vi "Main.Create XNET Data Sessions.vi"(6 "Data":T1 {"Outgoing"."Trigger.Refs"."Data Reference" format="%.0x"; "Outgoing"."Disable.Refs"."Data Reference" format="%.0x"; "Outgoing"."Data.Refs"."Data Reference" format="%.0x"; "Incoming"."Timing.Refs"."Data Reference" format="%.0x"; "Incoming"."Data.Refs"."Data Reference" format="%.0x"}, 8 "error in (no error)":errorcluster, 9 "Network":T16 {"Name" format="%.0x"}, 10 "J1939 XNET Settings":T17 {"Termination" items=["Off", "On"]}, 11 "DataTableLUT":variant) -> (0 "error out":errorcluster, 2 "XNET Sessions":T18 {"Outgoing.Frames.CountersAndProtections"."Protection Configurations"."CRC Channels"."Data Type" items=["Signed", "Unsigned", "IEEE Float"]; "Trigger.Refs"."Data Reference" format="%.0x"; "Disable.Refs"."Data Reference" format="%.0x"; "Timing.Refs"."Data Reference" format="%.0x"; "Network"."Name" format="%.0x"; "Incoming.Refs"."Data Reference" format="%.0x"; "Outgoing.Refs"."Data Reference" format="%.0x"}, 3 "DataTableLUT":variant)   [LabVIEW 2021, in "J1939 Addon Engine.lvlib"]
uses:
  J1939 Addon Engine.lvlib
  Types/Protocol.XNET Refs.ctl
  Addon Shared/Types/Monitor Settings.ctl
  <vilib>/NI VeriStand/Custom Device API/Block Data Reference.ctl
  <vilib>/NI VeriStand/Custom Device API/Data Reference.ctl
  Types/Main.Outgoing.Frame.Settings.ctl
  Addon Shared/Types/Outgoing Event Trigger Types.ctl
  SubModules/Frame-Protection-Support/Source/Shared/Types/Exported Frame Settings.ctl
  SubModules/Frame-Protection-Support/Source/Shared/Types/Exported Frame Type.ctl
  SubModules/Frame-Protection-Support/Source/Shared/Types/Exported Protection Settings.ctl
  SubModules/Frame-Protection-Support/Source/Shared/Types/Protection Type.ctl
  SubModules/Frame-Protection-Support/Source/Shared/Types/XNET Signal Configuration.ctl
  SubModules/Frame-Protection-Support/Source/Shared/Types/Exported Counter Settings.ctl
  SubModules/Frame-Protection-Support/Source/Shared/Types/Exported Event Trigger Type.ctl
  Addon Shared/Types/XNET Settings.ctl
  Addon Shared/Types/Device Settings.ctl
  Addon Shared/Types/Incoming Settings.ctl
  Addon Shared/Types/Incoming Frame Settings.ctl
  Addon Shared/Types/Outgoing Settings.ctl
  Addon Shared/Types/Outgoing Frame Settings.ctl
  <vilib>/xnet/xnet.llb/XNET Control Scope.ctl
  Support Libraries/J1939 Utilities/SubVIs/Convert CAN Arb ID to J1939 ID.vi
  <vilib>/xnet/xnet.llb/XNET Create Session (Signal Input Single-point).vi
  <vilib>/xnet/xnet.llb/XNET Create Session (Signal Output Single-point).vi
  <resource>/objmgr/xnet.rc
  <vilib>/NI VeriStand/Custom Device API/Custom Device API.lvlib
  Addon Shared/J1939 Addon Shared.lvlib
  SubModules/Frame-Protection-Support/Source/Shared/Protection and Counter Support Shared.lvlib
  Support Libraries/J1939 Utilities/J1939 Utilities.lvlib
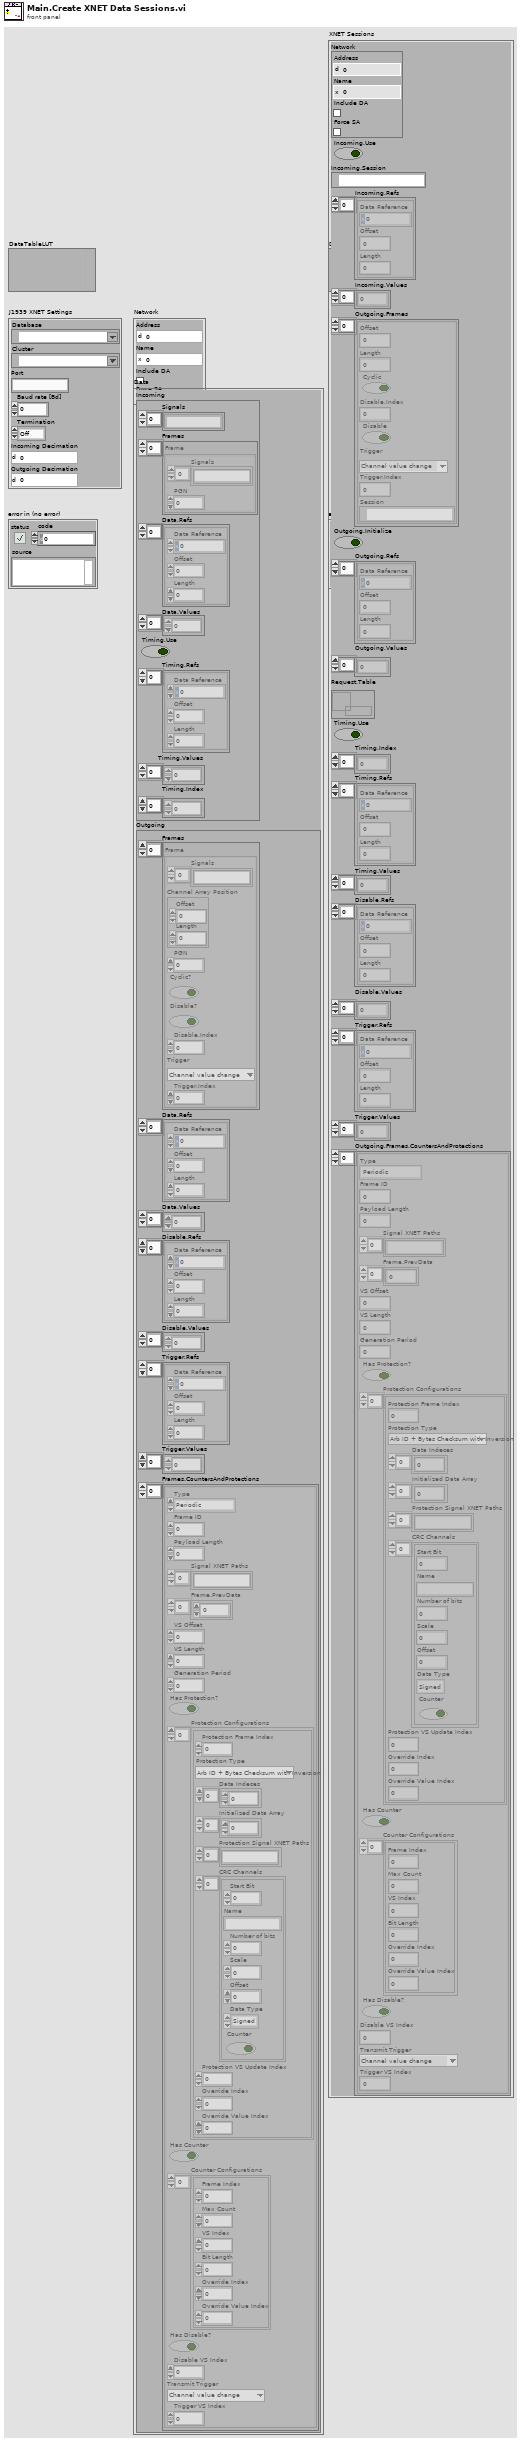
[diagram p1: front panel]
types:
  T1 = typedef "J1939 Addon Shared.lvlib/Device Settings.ctl" = cluster{"Incoming":T2, "Outgoing":T6}
  T2 = typedef "J1939 Addon Shared.lvlib/Incoming Settings.ctl" = cluster{"Signals":string[], "Frames":T3[], "Data.Refs":T4[], "Data.Values":dbl[], "Timing.Use":bool, "Timing.Refs":T4[], "Timing.Values":dbl[], "Timing.Index":i32[]}
  T3 = typedef "J1939 Addon Shared.lvlib/Incoming Frame Settings.ctl" = cluster{"Signals":string[], "PGN":u32}
  T4 = typedef "Custom Device API.lvlib/Block Data Reference.ctl" = cluster{"Data Reference":T5, "Offset":u64, "Length":u64}
  T5 = typedef "Custom Device API.lvlib/Data Reference.ctl" = i32
  T6 = typedef "J1939 Addon Shared.lvlib/Outgoing Settings.ctl" = cluster{"Frames":T7[], "Data.Refs":T4[], "Data.Values":dbl[], "Disable.Refs":T4[], "Disable.Values":dbl[], "Trigger.Refs":T4[], "Trigger.Values":dbl[], "Frames.CountersAndProtections":T9[]}
  T7 = typedef "J1939 Addon Shared.lvlib/Outgoing Frame Settings.ctl" = cluster{"Signals":string[], "Channel Array Position":cluster{"Offset":u32, "Length":u32}, "PGN":u32, "Cyclic?":bool, "Disable?":bool, "Disable.Index":i32, "Trigger":T8, "Trigger.Index":i32}
  T8 = typedef "J1939 Addon Shared.lvlib/Outgoing Event Trigger Types.ctl" = enum16{"Channel value change", "Trigger channel (not zero)", "Channel value change or trigger channel (not zero)", "Trigger channel (any value change)", "Channel value change or trigger channel (any value change)"}
  T9 = typedef "Protection and Counter Support Shared.lvlib/Exported Frame Settings.ctl" = cluster{"Type":T10, "Frame ID":u32, "Payload Length":u32, "Signal XNET Paths":string[], "Frame.PrevData":dbl[], "VS Offset":i32, "VS Length":i32, "Generation Period":u32, "Has Protection?":bool, "Protection Configurations":T11[], "Has Counter":bool, "Counter Configurations":T14[], "Has Disable?":bool, "Disable VS Index":i32, "Transmit Trigger":T15, "Trigger VS Index":i32}
  T10 = typedef "Protection and Counter Support Shared.lvlib/Exported Frame Type.ctl" = enum16{"Periodic", "Event", "Periodic/Event"}
  T11 = typedef "Protection and Counter Support Shared.lvlib/Exported Protection Settings.ctl" = cluster{"Protection Frame Index":i32, "Protection Type":T12, "Data Indeces":i32[], "Initialized Data Array":dbl[], "Protection Signal XNET Paths":string[], "CRC Channels":T13[], "Protection VS Update Index":i32, "Override Index":i32, "Override Value Index":i32}
  T12 = typedef "Protection and Counter Support Shared.lvlib/Protection Type.ctl" = enum16{"Arb ID + Bytes Checksum with Inversion", "Arb ID + Bytes CRC with Inversion", "Reversed Raw Signal Checksum with Inversion", "Concatenated Two's Compliment"}
  T13 = typedef "Protection and Counter Support Shared.lvlib/XNET Signal Configuration.ctl" = cluster{"Start Bit":i32, "Name":string, "Number of bits":i32, "Scale":dbl, "Offset":dbl, "Data Type":u32, "Counter":bool}
  T14 = typedef "Protection and Counter Support Shared.lvlib/Exported Counter Settings.ctl" = cluster{"Frame Index":i32, "Max Count":dbl, "VS Index":i32, "Bit Length":i64, "Override Index":i32, "Override Value Index":i32}
  T15 = typedef "Protection and Counter Support Shared.lvlib/Exported Event Trigger Type.ctl" = enum16{"Channel value change", "Trigger channel (not zero)", "Channel value change or trigger channel (not zero)", "Trigger channel (any value change)", "Channel value change or trigger channel (any value change)"}
  T16 = typedef "J1939 Addon Shared.lvlib/Monitor Settings.ctl" = cluster{"Address":u8, "Name":u64, "Include DA":bool, "Force SA":bool}
  T17 = typedef "J1939 Addon Shared.lvlib/XNET Settings.ctl" = cluster{"Database":refnum<k21>, "Cluster":refnum<k21>, "Port":string, "Baud rate [Bd]":u32, "Termination":u32, "Incoming Decimation":u32, "Outgoing Decimation":u32}
  T18 = typedef "J1939 Addon Engine.lvlib/Protocol.XNET Refs.ctl" = cluster{"Network":T16, "Incoming.Use":bool, "Incoming.Session":refnum<k21>, "Incoming.Refs":T4[], "Incoming.Values":dbl[], "Outgoing.Frames":T19[], "Outgoing.Initialize":bool, "Outgoing.Refs":T4[], "Outgoing.Values":dbl[], "Request.Table":refnum<k33>, "Timing.Use":bool, "Timing.Index":i32[], "Timing.Refs":T4[], "Timing.Values":dbl[], "Disable.Refs":T4[], "Disable.Values":dbl[], "Trigger.Refs":T4[], "Trigger.Values":dbl[], "Outgoing.Frames.CountersAndProtections":T9[]}
  T19 = typedef "J1939 Addon Engine.lvlib/Main.Outgoing.Frame.Settings.ctl" = cluster{"Offset":u32, "Length":u32, "Cyclic":bool, "Disable.Index":i32, "Disable":bool, "Trigger":T8, "Trigger.Index":i32, "Session":refnum<k21>}
  T20 = cluster{"read mode":enum16{"polling", "blocking"}, "write mode":enum16{"polling", "blocking"}}
  T21 = typedef "XNET Control Scope.ctl" = u32
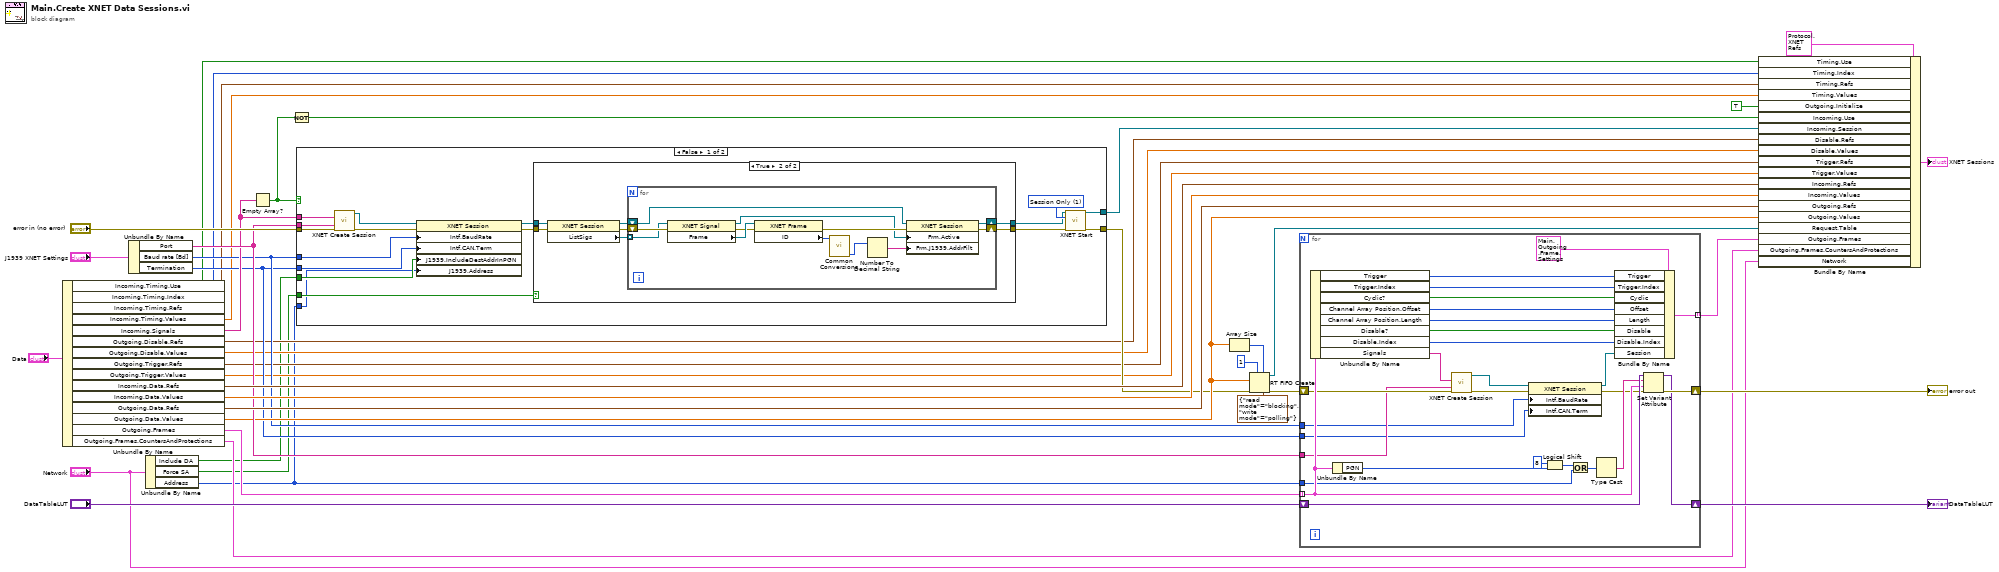
[diagram p0: block diagram]
diagram:
  n1 = Unbundle By Name("Data") -> ("Incoming.Timing.Use"=w10:bool, "Incoming.Timing.Index"=w11:i32[], "Incoming.Timing.Refs"=w12:T4[], "Incoming.Timing.Values"=w13:dbl[], "Incoming.Signals"=w29:string[], "Outgoing.Disable.Refs"=w6:T4[], "Outgoing.Disable.Values"=w5:dbl[], "Outgoing.Trigger.Refs"=w8:T4[], "Outgoing.Trigger.Values"=w7:dbl[], "Incoming.Data.Refs"=w33:T4[], "Incoming.Data.Values"=w32:dbl[], "Outgoing.Data.Refs"=w31:T4[], "Outgoing.Data.Values"=w24:dbl[], "Outgoing.Frames"=w34:T7[], "Outgoing.Frames.CountersAndProtections"=w4:T9[])
  n2 = Unbundle By Name("J1939 XNET Settings") -> ("Port"=w30:string, "Baud rate [Bd]"=w17:u32, "Termination"=w16:u32)
  n3 = Unbundle By Name("Network") -> ("Include DA"=w3:bool, "Force SA"=w2:bool, "Address"=w1:u8)
  n4 = Empty Array?(array=w29) -> (empty?=w28:bool)
  n5 = Not(x=w28) -> (.not. x?=w27:bool)
  n6 = case shown="False" w28 {
    tunnel: [w49 _] -> w14
    tunnel: "error in (no error)" -> [w58 w80]
    tunnel: [w50 w80] -> w19
    tunnel: w30 -> [w57 _]
    tunnel: w29 -> [w56 _]
    tunnel: w17 -> [w52 _]
    tunnel: w16 -> [w51 _]
    tunnel: w3 -> [w48 _]
    tunnel: w2 -> [w43 _]
    tunnel: w1 -> [w42 _]
    frame False {
      w55 = T21 1 items=["Normal", "Session Only", "Interface Only", "Session Only Blocking"] ("scope (normal)")
      n7 = call-poly <vilib>:"XNET Create Session.vi"("signal list"=w56, "interface"=w57, "error in (no error)"=w58) -> ("session out"=w53:refnum<k21>, "error out"=w54:errorcluster)  [unwired: 11 in]
      n8 = property class="XNET Session"(reference=w53, error in=w54, "Intf.BaudRate"=w52, "Intf.CAN.Term"=w51, "J1939.IncludeDestAddrInPGN"=w48, "J1939.Address"=w42) -> (reference out=w46:refnum<k21>, error out=w47:errorcluster)
      n9 = case shown="True" w43 {
        tunnel: w47 -> [w60 w67]
        tunnel: w46 -> [w59 w66]
        tunnel: [w60 w62] -> w45
        tunnel: [w59 w61] -> w44
        frame False {
        }
        frame True {
          n10 = property class="XNET Session"(reference=w66, error in=w67) -> (reference out=w63:refnum<k21>, error out=w65:errorcluster, "ListSigs"=w64:refnum<k21>[])
          n11 = for {
            shift-right: [w78] -> w61
            shift-left: w63 -> [w79]
            shift-right: [w77] -> w62
            shift-left: w65 -> [w74]
            tunnel: w64 -> [w71] mode=indexing
            n12 = property class="XNET Signal"(reference=w71, error in=w74) -> (reference out=w70:refnum<k21>, error out=w73:errorcluster, "Frame"=w75:refnum<k21>)
            n13 = property class="XNET Frame"(reference=w75, error in=w73) -> (error out=w72:errorcluster, "ID"=w69:u32)  [unwired: 1 out]
            n14 = call-poly "Common Conversions.vi"("Arb ID"=w69) -> ("Source Address"=w68:u8)  [unwired: 11 in, 3 out]
            n15 = Number To Decimal String(number=w68) -> (decimal integer string=w76:string)  [unwired: 1 in]
            n16 = property class="XNET Session"(reference=w79, error in=w72, "Frm.Active"=w70, "Frm.J1939.AddrFilt"=w76) -> (reference out=w78:refnum<k21>, error out=w77:errorcluster)
          }
        }
      }
      n17 = call <vilib>:"XNET Start.vi"("session in"=w44, "scope (normal)"=w55, "error in (no error)"=w45) -> ("session out"=w49:refnum<k21>, "error out"=w50:errorcluster)  [unwired: 11 in]
    }
    frame True {
    }
  }
  n18 = Array Size(array=w24) -> (size(s)=w23:i32)
  n19 = RT FIFO Create(1:w24, 3:w19, 4:1 ("max queue size (-1, unlimited)"), 6:w23, 7:T20 {"read mode"=enum."blocking", "write mode"=enum."polling"} ("r/w modes (polling,polling)")) -> (8:w20:refnum<k33>, 11:w25:errorcluster)  [unwired: 3 in, 1 out]
  n20 = for {
    tunnel: w34 -> [w100] mode=indexing
    tunnel: w1 -> [w96]
    shift-right: [w101] -> w41
    shift-left: "DataTableLUT" -> [w104]
    shift-right: [w102] -> w18
    shift-left: w25 -> [w99]
    tunnel: w30 -> [w98]
    tunnel: w17 -> [w93]
    tunnel: w16 -> [w92]
    tunnel: [w86] -> w9 mode=indexing
    n21 = Unbundle By Name(w100) -> ("Trigger"=w82:T8, "Trigger.Index"=w83:i32, "Cyclic?"=w89:bool, "Channel Array Position.Offset"=w88:u32, "Channel Array Position.Length"=w87:u32, "Disable?"=w85:bool, "Disable.Index"=w84:i32, "Signals"=w97:string[])
    n22 = Unbundle By Name(w100) -> ("PGN"=w108:u32)
    n23 = call-poly <vilib>:"XNET Create Session.vi"("signal list"=w97, "interface"=w98, "error in (no error)"=w99) -> ("session out"=w94:refnum<k21>, "error out"=w95:errorcluster)  [unwired: 11 in]
    n24 = property class="XNET Session"(reference=w94, error in=w95, "Intf.BaudRate"=w93, "Intf.CAN.Term"=w92) -> (reference out=w81:refnum<k21>, error out=w91:errorcluster)
    n25 = Logical Shift(y=i16 8, x=w108) -> (x << y=w106:u32)
    n26 = Or(x=w106, y=w96) -> (x .or. y?=w105:u32)
    n27 = Type Cast(x=w105) -> (*(type *) &x=w103:string)  [unwired: 1 in]
    n28 = Bundle By Name(cluster=T19 {"Offset"=0, "Length"=0, "Cyclic"=FALSE, "Disable.Index"=0, "Disable"=FALSE, "Trigger"=enum."Channel value change", "Trigger.Index"=0, "Session"=""} ("Channel Array Position"), "Trigger"=w82, "Trigger.Index"=w83, "Cyclic"=w89, "Offset"=w88, "Length"=w87, "Disable"=w85, "Disable.Index"=w84, "Session"=w81) -> (w86:T19)
    n29 = Set Variant Attribute(Variant=w104, name=w103, value=w100, error in=w91) -> (Variant out=w101:variant, error out=w102:errorcluster)  [unwired: 1 out]
  }
  "error out" <- w18
  "DataTableLUT" <- w41
  n30 = Bundle By Name(cluster=T18 {"Network"={"Address"=0, "Name"=0, "Include DA"=FALSE, "Force SA"=FALSE}, "Incoming.Use"=FALSE, "Incoming.Session"="", "Incoming.Refs"=[], "Incoming.Values"=[], "Outgoing.Frames"=[], "Outgoing.Initialize"=FALSE, "Outgoing.Refs"=[], "Outgoing.Values"=[], "Request.Table"=refnum, "Timing.Use"=FALSE, "Timing.Index"=[], "Timing.Refs"=[], "Timing.Values"=[], "Disable.Refs"=[], "Disable.Values"=[], "Trigger.Refs"=[], "Trigger.Values"=[], "Outgoing.Frames.CountersAndProtections"=[]}, "Timing.Use"=w10, "Timing.Index"=w11, "Timing.Refs"=w12, "Timing.Values"=w13, "Outgoing.Initialize"=TRUE ("Initialize Outgoing?"), "Incoming.Use"=w27, "Incoming.Session"=w14, "Disable.Refs"=w6, "Disable.Values"=w5, "Trigger.Refs"=w8, "Trigger.Values"=w7, "Incoming.Refs"=w33, "Incoming.Values"=w32, "Outgoing.Refs"=w31, "Outgoing.Values"=w24, "Request.Table"=w20, "Outgoing.Frames"=w9, "Outgoing.Frames.CountersAndProtections"=w4, "Network"="Network") -> (→"XNET Sessions":T18)
